vi "test_OpenClose (Multi Sessions).vi"() -> ()   [LabVIEW 2020]
uses:
  <instrlib>/AIM GmbH/_AIM 664/bsp/Fdx Create Session (RX-Monitor).vi
  <instrlib>/AIM GmbH/_AIM 664/bsp/Fdx Create Session (Tx-Generic).vi
  <instrlib>/AIM GmbH/_AIM 664/bsp/Fdx Create Session (Rx-VL-Oriented).vi
  <instrlib>/AIM GmbH/_AIM 664/AIM664LV.lvlib
  <instrlib>/AIM GmbH/_AIM 664/bsp/Fdx Create Session (Tx-UDP Port-Oriented).vi
panel:
  in  "simulate execution time mS":u32=10
  out "executed":i32
  in  "Iterations":i32=1
  in  "idle before iterations mS":u32=1000
  in  "board 2":u32
  in  "port 2":u32=1
  out "error out 2":errorcluster caption="error out"
  out "error out":errorcluster
  in  "port":u32
  in  "board":u32
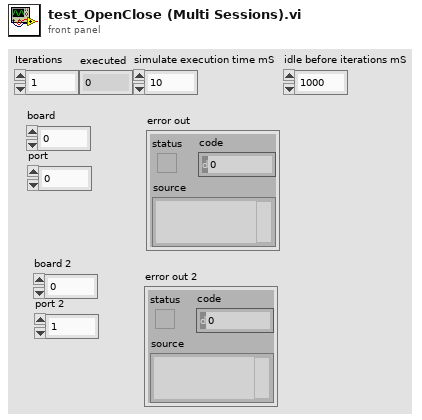
[diagram p1: front panel]
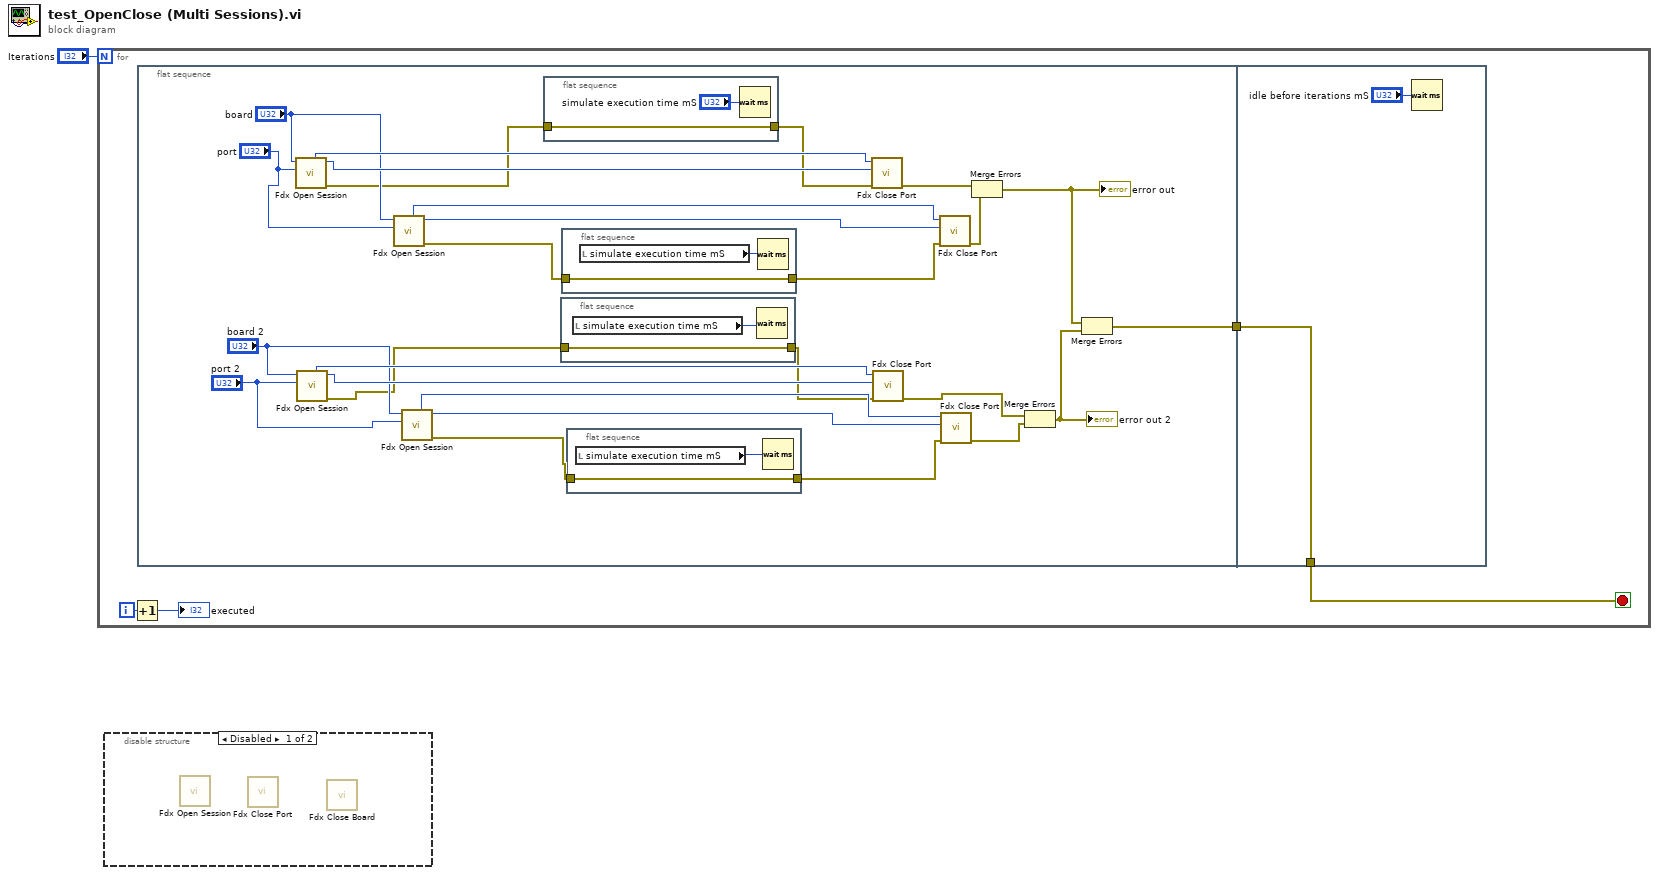
[diagram p0: block diagram]
diagram:
  n1 = for {
    N: "Iterations" -> [_]
    i -> [w3]
    stop <- w5 stop-if-true
    n2 = Increment(x=w3) -> (x+1=→"executed":i32)
    n3 = flat-sequence {
      tunnel: [w14] -> w4
      tunnel: [w41] -> w5
      tunnel: w4 -> [w41]
      frame #0 {
        n4 = call-poly <instrlib>:"Fdx Open Session.vi"("port"="port", "board"="board") -> ("error out"=w13:errorcluster, "port handle out"=w32:u32, "InstrumentHandle_board out"=w31:u32)  [unwired: 4 in, 3 out]
        n5 = call-poly <instrlib>:"Fdx Open Session.vi"("port"="port 2", "board"="board 2") -> ("error out"=w9:errorcluster, "port handle out"=w29:u32, "InstrumentHandle_board out"=w30:u32)  [unwired: 4 in, 3 out]
        n6 = call-poly <instrlib>:"Fdx Open Session.vi"("port"="port", "board"="board") -> ("error out"=w11:errorcluster, "InstrumentHandle_port out"=w26:u32, "InstrumentHandle_board out"=w25:u32)  [unwired: 4 in, 3 out]
        n7 = call-poly <instrlib>:"Fdx Open Session.vi"("port"="port 2", "board"="board 2") -> ("error out"=w7:errorcluster, "InstrumentHandle_port out"=w22:u32, "InstrumentHandle_board out"=w21:u32)  [unwired: 4 in, 3 out]
        n8 = flat-sequence {
          tunnel: w13 -> [w40]
          tunnel: [w40] -> w12
          frame #0 {
            n9 = Wait (ms)(milliseconds to wait="simulate execution time mS") -> ()  [unwired: 1 out]
          }
        }
        n10 = flat-sequence {
          tunnel: w9 -> [w36]
          tunnel: [w36] -> w8
          frame #0 {
            n11 = local read "simulate execution time mS"() -> (w35:u32)
            n12 = Wait (ms)(milliseconds to wait=w35) -> ()  [unwired: 1 out]
          }
        }
        n13 = flat-sequence {
          tunnel: w11 -> [w38]
          tunnel: [w38] -> w10
          frame #0 {
            n14 = local read "simulate execution time mS"() -> (w37:u32)
            n15 = Wait (ms)(milliseconds to wait=w37) -> ()  [unwired: 1 out]
          }
        }
        n16 = flat-sequence {
          tunnel: w7 -> [w34]
          tunnel: [w34] -> w6
          frame #0 {
            n17 = local read "simulate execution time mS"() -> (w33:u32)
            n18 = Wait (ms)(milliseconds to wait=w33) -> ()  [unwired: 1 out]
          }
        }
        n19 = call <instrlib>:"Fdx Close Port.vi"("error in"=w12, "InstrumentHandle_port in"=w32, "InstrumentHandle_board in"=w31) -> ("error out"=w20:errorcluster)  [unwired: 7 in, 1 out]
        n20 = call <instrlib>:"Fdx Close Port.vi"("error in"=w8, "InstrumentHandle_port in"=w29, "InstrumentHandle_board in"=w30) -> ("error out"=w17:errorcluster)  [unwired: 7 in, 1 out]
        n21 = call <instrlib>:"Fdx Close Port.vi"("error in"=w10, "InstrumentHandle_port in"=w26, "InstrumentHandle_board in"=w25) -> ("error out"=w19:errorcluster)  [unwired: 7 in, 1 out]
        n22 = call <instrlib>:"Fdx Close Port.vi"("error in"=w6, "InstrumentHandle_port in"=w22, "InstrumentHandle_board in"=w21) -> ("error out"=w18:errorcluster)  [unwired: 7 in, 1 out]
        n23 = Merge Errors(w20, w19) -> (w16:errorcluster)
        "error out" <- w16
        n24 = Merge Errors(w17, w18) -> (w15:errorcluster)
        "error out 2" <- w15
        n25 = Merge Errors(w16, w15) -> (w14:errorcluster)
      }
      frame #1 {
        n26 = Wait (ms)(milliseconds to wait="idle before iterations mS") -> ()  [unwired: 1 out]
      }
    }
  }
  n27 = disable-structure shown="Disabled" {
    frame Disabled {
      n28 = call-poly <instrlib>:"Fdx Open Session.vi"() -> ()  [unwired: 7 in, 5 out]
      n29 = call <instrlib>:"Fdx Close Port.vi"() -> ()  [unwired: 10 in, 2 out]
      n30 = call <instrlib>:"Fdx Close Board.vi"() -> ()  [unwired: 11 in, 1 out]
    }
    frame Enabled {
    }
  }
